vi "getStagePositionStatus.vi"(8 "error in (no error)":errorcluster, 9 "Stage Position (mm)":dbl, 11 "Microscope in":refnum<class "Microscope.lvclass">) -> (0 "error out":errorcluster, 2 "stage position ok":bool, 3 "Microscope out":refnum<class "Microscope.lvclass">)   [LabVIEW 2012, in "Microscope.lvclass"]
doc: "Outputs true if stage position is greater than end position (forward).\nOutputs true if stage position is lesser than end position (backward)."
uses:
  classes/Microscope.lvclass
  classes/Microscope.lvclass/Microscope.ctl
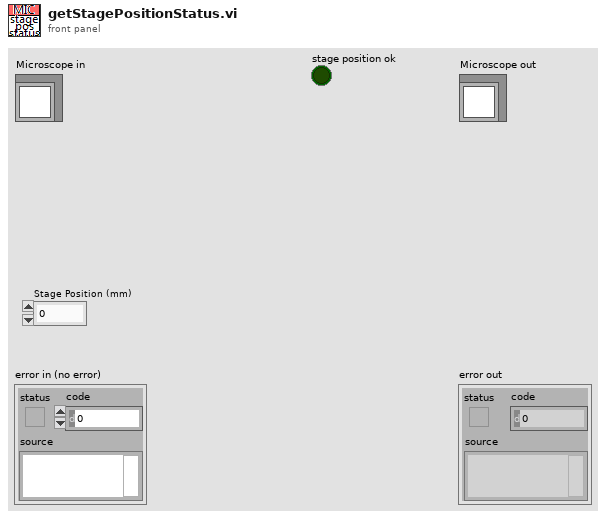
[diagram p1: front panel]
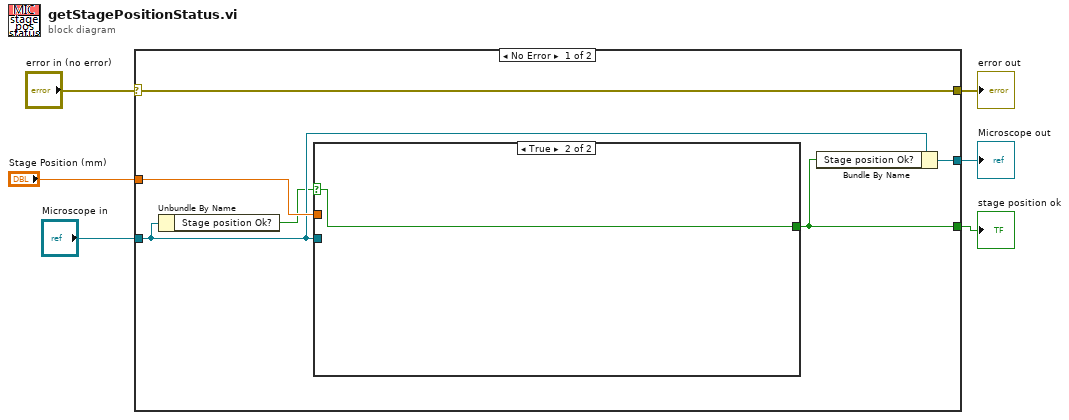
[diagram p0: block diagram]
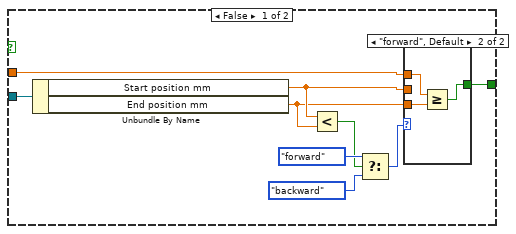
[diagram p2: hidden frame]
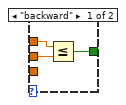
[diagram p3: hidden frame]
diagram:
  n1 = case shown="No Error" "error in (no error)" {
    selector: "error in (no error)" -> [w11 w30]
    tunnel: [w11 w30] -> w5
    tunnel: [w8 w29] -> w3
    tunnel: "Microscope in" -> [w9 w29]
    tunnel: [w12 _] -> w2
    tunnel: "Stage Position (mm)" -> [w10 _]
    frame No Error {
      n2 = Unbundle By Name(w9) -> ("Stage position Ok?"=w7:bool)
      n3 = case shown="True" w7 {
        selector: w7 -> [_ w28]
        tunnel: w9 -> [w21 _]
        tunnel: w10 -> [w14 _]
        tunnel: [w13 w28] -> w12
        frame False {
          n4 = Unbundle By Name(w21) -> ("Start position mm"=w16:dbl, "End position mm"=w15:dbl)
          n5 = Less?(x=w16, y=w15) -> (x < y?=w18:bool)
          n6 = Select(t=enum16{"", "forward", "backward"}."forward", s=w18, f=enum16{"", "forward", "backward"}."backward") -> (s? t:f=w17:enum16{"", "forward", "backward"})
          n7 = case shown="\"forward\", Default" w17 {
            tunnel: w15 -> [_ w27]
            tunnel: [w24 w26] -> w13
            tunnel: w14 -> [w23 w25]
            tunnel: w16 -> [w22 _]
            frame "backward" {
              n8 = Less Or Equal?(x=w23, y=w22) -> (x <= y?=w24:bool)
            }
            frame "forward", Default {
              n9 = Greater Or Equal?(x=w25, y=w27) -> (x >= y?=w26:bool)
            }
          }
        }
        frame True {
        }
      }
      n10 = Bundle By Name(cluster=w9, "Stage position Ok?"=w12) -> (w8:refnum<class "Microscope.lvclass">)
    }
    frame Error {
    }
  }
  "error out" <- w5
  "Microscope out" <- w3
  "stage position ok" <- w2
